vi "Release Notifiers.vi"(8 "error in":errorcluster) -> (0 "error out":errorcluster)   [LabVIEW 2019]
doc: "Release all queues\n\n-----\nJuan Navarro\nLab it Studio"
uses:
  Sequencer/Sequencer Handshake.lvlib
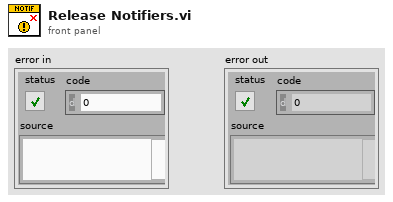
[diagram p1: front panel]
types:
  T1 = enum16{"Obtain", "Send", "Get Notifier", "Release"}
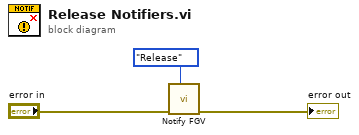
[diagram p0: block diagram]
diagram:
  n1 = call "Notify FGV.vi"("Actions"=T1."Release", "error in"="error in") -> ("error out"=→"error out":errorcluster)  [unwired: 8 in, 1 out]
